vi "ImageReadImage.vi"   [LabVIEW 2012, in "Image.lvclass"]
uses:
  classes/Image.lvclass
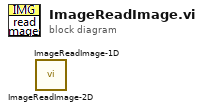
[diagram p0: block diagram]
diagram:
  n1 = call "ImageReadImage-2D.vi"() -> ()  [unwired: 9 in, 3 out]
  n2 = call "ImageReadImage-1D.vi"() -> ()  [unwired: 9 in, 3 out]
